vi "Error Query.vi"(0 "VISA Resource Name":refnum<visa-resource-name>, 11 "error in (no error)":errorcluster) -> (4 "VISA Resource Name Out":refnum<visa-resource-name>, 8 "Error":i32, 10 "Error Message":string, 15 "error out":errorcluster)   [LabVIEW 2018, in "Agilent PNA Series.lvlib"]
doc: "This VI reads an error from the instrument. It expects to see errors in SCPI format (#,\"error message\"). If an error query is not supported, it returns a warning."
uses:
  Agilent PNA Series.lvlib
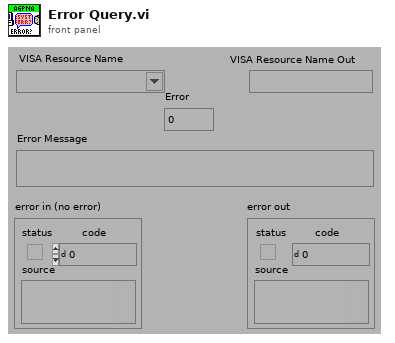
[diagram p1: front panel]
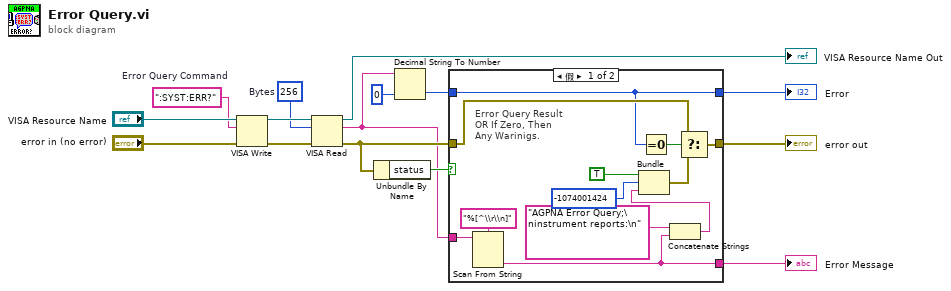
[diagram p0: block diagram]
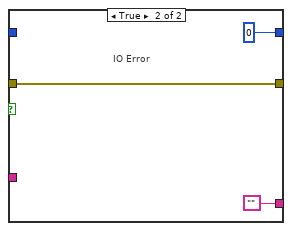
[diagram p2: hidden frame]
diagram:
  w7 = u32 256  # Bytes
  w5 = ":SYST:ERR?"  # Error Query Command
  n1 = VISA Write(VISA resource name="VISA Resource Name", write buffer=w5, error in (no error)="error in (no error)") -> (VISA resource name out=w8:refnum<visa-resource-name>, error out=w6:errorcluster)  [unwired: 1 out]
  n2 = VISA Read(VISA resource name=w8, byte count=w7, error in (no error)=w6) -> (VISA resource name out=→"VISA Resource Name Out":refnum<visa-resource-name>, read buffer=w3:string, error out=w9:errorcluster)  [unwired: 1 out]
  n3 = Unbundle By Name(w9) -> ("status"=w4:bool)
  n4 = Decimal String To Number(string=w3, default (0L)=0) -> (number=w1:i32)  [unwired: 1 in, 1 out]
  n5 = case shown="假" w4 {
    tunnel: w3 -> [w18 _]
    tunnel: w9 -> [w22 w30]
    tunnel: [w23 w30] -> w10
    tunnel: [w16 ""] -> w15
    tunnel: [w19 0] -> w14
    tunnel: w1 -> [w19 _]
    frame False {
      # "Error Query Result\nOR If Zero, Then\nAny Warinigs."
      n6 = Scan From String(format string="%[^\\r\\n]", input string=w18) -> (output 1=w16:string)  [unwired: 3 in, 3 out]
      n7 = Equal To 0?(x=w19) -> (x = 0?=w20:bool)
      n8 = Concatenate Strings("AGPNA Error Query;\ninstrument reports:\n" ("Source"), w16) -> (w25:string)
      n9 = Bundle("Status"=TRUE, "Code"=-1074001424, w25) -> (w24:cluster{"Status":bool, "Code":i32, string})  [unwired: 1 in]
      n10 = Select(t=w22, s=w20, f=w24) -> (s? t:f=w23:errorcluster)
    }
    frame True {
      # "IO Error"
    }
  }
  "Error Message" <- w15
  "Error" <- w14
  "error out" <- w10
